vi "웹서버 온도 통신 연결.vi"() -> ()   [LabVIEW 2019]
uses:
  <vilib>/httpClient/ClientHandle.ctl
  <vilib>/DAQmx/read.llb/DAQmx Read (Analog 1D DBL 1Chan NSamp).vi
  <vilib>/Analysis/baseanly.llb/Mean (DBL).vi
  <vilib>/DAQmx/create/channels.llb/DAQmx Create Channel (AI-Temperature-Thermocouple).vi
  <vilib>/DAQmx/configure/timing.llb/DAQmx Timing (Sample Clock).vi
  <vilib>/DAQmx/miscellaneous.llb/DAQmx Fill In Error Info.vi
  <vilib>/httpClient/PUTBuffer.vi
  <vilib>/httpClient/LabVIEWHTTPClient.lvlib
  <vilib>/Analysis/NI_AALBase.lvlib
panel:
  out "JSON 문자열":string
  out "y":u32
  in  "불리언":bool
  out "숫자형":i32
  in  "physical channels":tag caption="물리적 채널"
  in  "thermocouple type":i32(ring)=10072 caption="열전쌍 타입" items=["J"=10072, "K"=10073, "N"=10077, "R"=10082, "S"=10085, "T"=10086, "B"=10047, "E"=10055]
  out "error out":errorcluster caption="에러 출력"
  in  "에러 입력(에러 없음)":errorcluster
  out "참조 번호 출력":T1 caption="client handle out"
  in  "참조 번호 입력":T1 caption="client handle out"
  out "body 3":string caption="웹서버에 입력된 문자열"
  out "headers 3":string caption="연결확인 메세지 출력"
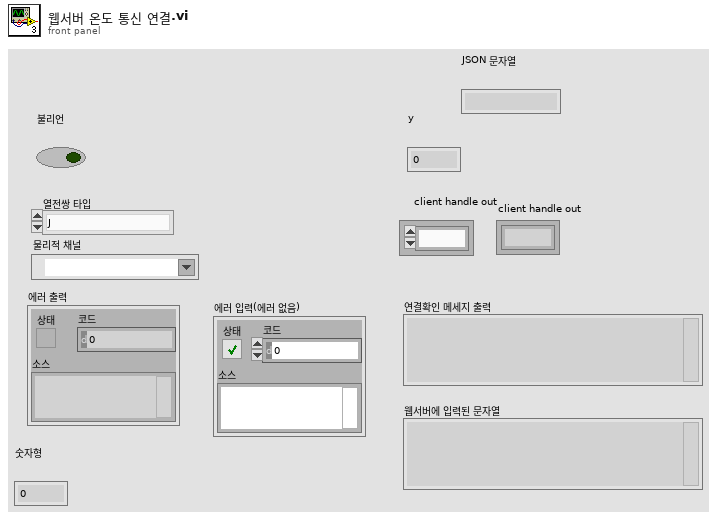
[diagram p1: front panel]
types:
  T1 = typedef "LabVIEWHTTPClient.lvlib/ClientHandle.ctl" = refnum<k1>
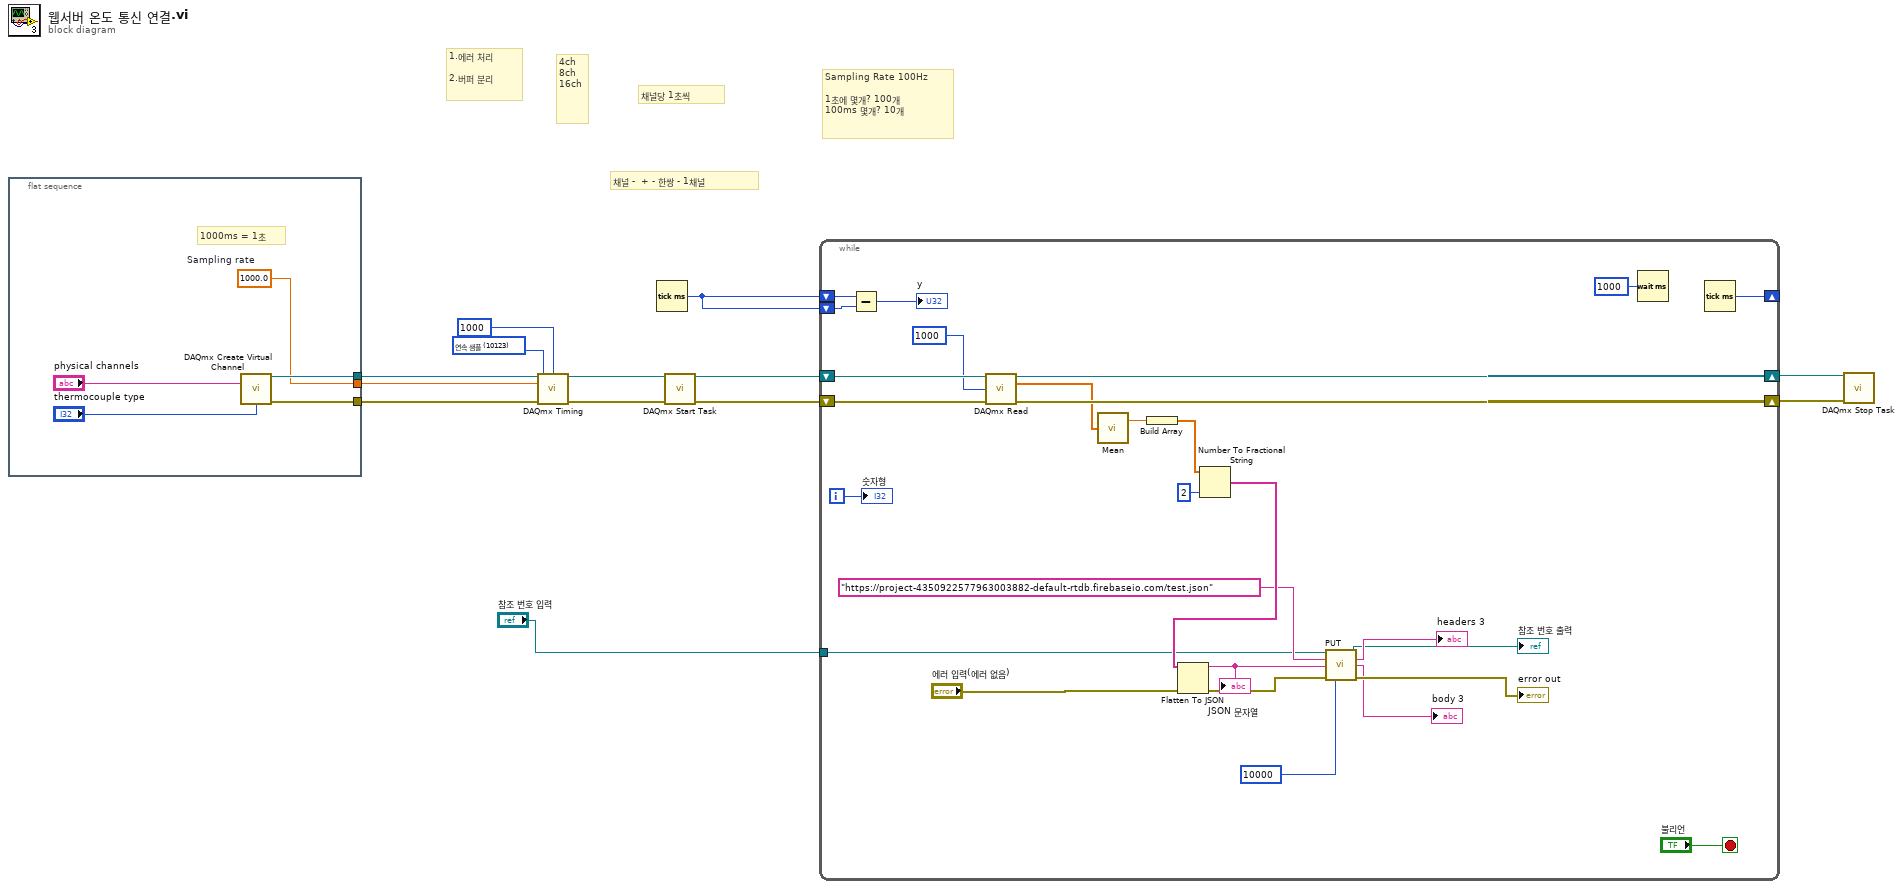
[diagram p0: block diagram]
diagram:
  w2 = 10123 items=["유한 샘플"=10178, "연속 샘플"=10123, "하드웨어 타이밍에 의한 단일 포인트"=12522] ("sample mode")
  # "1.에러 처리 \n\n2.버퍼 분리"
  # "채널 -  + - 한쌍 - 1채널"
  # "채널당 1초씩"
  # "4ch\n8ch\n16ch"
  # "Sampling Rate 100Hz\n\n1초에 몇개? 100개\n100ms 몇개? 10개"
  n1 = flat-sequence {
    tunnel: [w16] -> w8
    tunnel: [w15] -> w6
    tunnel: [w14] -> w3
    frame #0 {
      w14 = 1000.0  # Sampling rate
      # "1000ms = 1초"
      n2 = call-poly <vilib>:"DAQmx Create Virtual Channel.vi"("physical channels"="physical channels", "thermocouple type"="thermocouple type") -> ("task out"=w16:refnum<k21>, "error out"=w15:errorcluster)  [unwired: 12 in]
    }
  }
  n3 = call-poly <vilib>:"DAQmx Timing.vi"("task/channels in"=w8, "sample mode"=w2, "samples per channel"=1000, "rate"=w3, "error in"=w6) -> ("task out"=w7:refnum<k21>, "error out"=w5:errorcluster)  [unwired: 9 in]
  n4 = Tick Count (ms)() -> (millisecond timer value=w9:u32)
  n5 = call <vilib>:"DAQmx Start Task.vi"("task/channels in"=w7, "error in"=w5) -> ("task out"=w11:refnum<k21>, "error out"=w10:errorcluster)  [unwired: 12 in]
  n6 = while {
    shift-right: [w43] -> w13
    shift-left: w11 -> [w45]
    shift-right: [w42] -> w12
    shift-left: w10 -> [w44]
    shift-right: [w38] -> _
    shift-left: w9 -> [w37]
    shift-left: w9 -> [w36]
    tunnel: "참조 번호 입력" -> [w19]
    i -> [w41]
    stop <- "불리언" stop-if-true
    n7 = Subtract(x=w37, y=w36) -> (x-y=→"y":u32)
    n8 = call-poly <vilib>:"DAQmx Read.vi"("task/channels in"=w45, "number of samples per channel"=1000, "error in"=w44) -> ("task out"=w43:refnum<k21>, "data"=w33:dbl[], "error out"=w42:errorcluster)  [unwired: 10 in]
    n9 = call-poly <vilib>:"Mean.vi"("X"=w33) -> ("mean"=w32:dbl)  [unwired: 1 out]
    n10 = Build Array(w32) -> (w31:dbl[])
    n11 = Number To Fractional String(number=w31, precision (6)=i16 2 ("정밀도(6)")) -> (F-format string=w39:string[])  [unwired: 2 in]
    n12 = Flatten To JSON(anything=w39, error in (no error)="에러 입력(에러 없음)") -> (JSON string=w27:string, 11:w28:errorcluster)  [unwired: 1 in]
    "JSON 문자열" <- w27
    n13 = call-poly <vilib>:"PUT.vi"("client handle"=w19, "url"="https://project-4350922577963003882-default-rtdb.firebaseio.com/test.json", "buffer"=w27, "error in (no error)"=w28, "timeout (10000)"=10000) -> ("client handle out"=→"참조 번호 출력":T1, "headers"=→"headers 3":string, "body"=→"body 3":string, "error out"=→"error out":errorcluster)  [unwired: 7 in]
    n14 = Wait (ms)(milliseconds to wait=u32 1000 ("대기 시간 (ms)")) -> ()  [unwired: 1 out]
    n15 = Tick Count (ms)() -> (millisecond timer value=w38:u32)
    "숫자형" <- w41
  }
  n16 = call <vilib>:"DAQmx Stop Task.vi"("task/channels in"=w13, "error in"=w12) -> ()  [unwired: 12 in, 2 out]
